vi "AoC23-Read input file to 1D array str.vi"(11 "input file":path) -> (2 "input text":string, 3 "input":string[](array[string]))   [LabVIEW 2021]
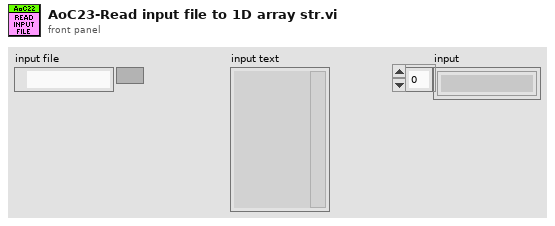
[diagram p1: front panel]
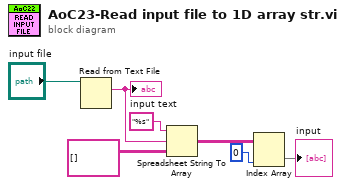
[diagram p0: block diagram]
diagram:
  n1 = Read from Text File(file (use dialog)="input file") -> (text=w6:string)  [unwired: 3 in, 3 out]
  "input text" <- w6
  n2 = Spreadsheet String To Array(format string="%s", spreadsheet string=w6, array type (2D Dbl)=string[][] []) -> (array=w3:string[][])  [unwired: 1 in]
  n3 = Index Array(array=w3, index (col)=0 ("disabled index (col)")) -> (element=→"input":string[])  [unwired: 1 in]
